vi "SubVI_AutoscaleSliderToImageSize.vi"(0 "X slider refnum in":refnum<vi>, 1 "Y slider refnum in":refnum<vi>, 2 "Image RefNum":T1) -> ()   [LabVIEW 2016]
uses:
  <vilib>/vision/Image Controls.llb/IMAQ Image.ctl
  <resource>/objmgr/IMAQImage.rc
panel:
  # "This subVI sets the maximum\nvalue of two sliders to match\nthe dimensions of the input\nimage."
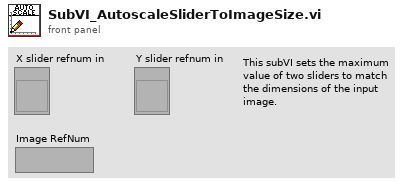
[diagram p1: front panel]
types:
  T1 = typedef "IMAQ Image.ctl" = refnum<image>
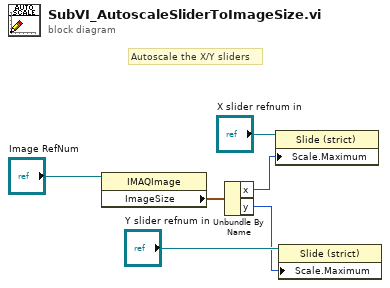
[diagram p0: block diagram]
diagram:
  # "Autoscale the X/Y sliders"
  n1 = property class="IMAQImage"(reference="Image RefNum") -> ("ImageSize"=w5:cluster{"x":i32, "y":i32})  [unwired: 1 in, 2 out]
  n2 = Unbundle By Name(w5) -> ("x"=w2:i32, "y"=w1:i32)
  n3 = property on="Property Node" class="Slide (strict)"(reference="X slider refnum in", "Scale.Maximum"=w2) -> ()  [unwired: 1 in, 2 out]
  n4 = property on="Property Node" class="Slide (strict)"(reference="Y slider refnum in", "Scale.Maximum"=w1) -> ()  [unwired: 1 in, 2 out]
